vi "Find free COM ports.vi"(11 "regular expression":string="COM[0-9]+") -> (3 "Free COM ports":string[](array[string]))   [LabVIEW 2021, in "MatS Libs.lvlib"]
doc: "Returns VISA aliases for free ports that matches a regular expresion.\nDefault regular expression is set to return free COM ports."
uses:
  <vilib>/Instr/_visa.llb/VISA Find Search Mode.ctl
  <userlib>/MatS Libs/MatS Libs.lvlib
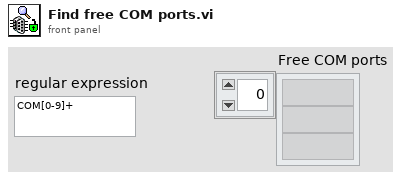
[diagram p1: front panel]
types:
  T1 = typedef "VISA Find Search Mode.ctl" = u32
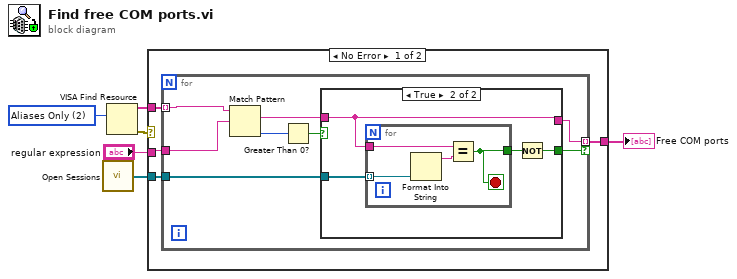
[diagram p0: block diagram]
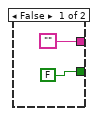
[diagram p2: hidden frame]
diagram:
  w4 = T1 2 items=["Canonical Names Only"=0, "Aliases Only"=2, "Include Matching Aliases"=3, "Include All Aliases"=4] ("Search Mode")
  n1 = call <vilib>:"Open Sessions.vi"() -> ("Array of Refnums"=w5:refnum<visa-resource-name>[])  [unwired: 2 in]
  n2 = VISA Find Resource(10:w4) -> (0:w1:errorcluster, 3:w3:string[])  [unwired: 2 in, 1 out]
  n3 = case shown="No Error" w1 {
    tunnel: [w10 _] -> w6
    tunnel: w5 -> [w9 _]
    tunnel: w3 -> [w8 _]
    tunnel: "regular expression" -> [w7 _]
    frame No Error {
      n4 = for {
        tunnel: w8 -> [w18] mode=indexing
        tunnel: w9 -> [w14]
        tunnel: [w13] -> w10 mode=indexing if=w12
        tunnel: w7 -> [w11]
        n5 = Match Pattern(string=w18, regular expression=w11) -> (match substring=w15:string, offset past match=w17:i32)  [unwired: 1 in, 2 out]
        n6 = Greater Than 0?(x=w17) -> (x > 0?=w16:bool)
        n7 = case shown="True" w16 {
          tunnel: w15 -> [_ w21]
          tunnel: w14 -> [_ w24]
          tunnel: [FALSE w22] -> w12
          tunnel: ["" ("String") w21] -> w13
          frame False {
          }
          frame True {
            n8 = for {
              tunnel: w24 -> [w28] mode=indexing
              tunnel: w21 -> [w26]
              tunnel: [w27] -> w23
              stop <- w27 stop-if-true
              n9 = Format Into String(w28) -> (resulting string=w25:string)  [unwired: 3 in, 1 out]
              n10 = Equal?(x=w26, y=w25) -> (x = y?=w27:bool)
            }
            n11 = Not(x=w23) -> (.not. x?=w22:bool)
          }
        }
      }
    }
    frame Error {
    }
  }
  "Free COM ports" <- w6
